vi "GetRotaryColorScaleReference.vi"(8 "error in":errorcluster, 11 "RotaryColorScale in":refnum<class "RotaryColorScale.lvclass">) -> (0 "error out":errorcluster, 1 "color scale reference":refnum<vi>, 3 "RotaryColorScale out":refnum<class "RotaryColorScale.lvclass">)   [LabVIEW 2014, in "Raspberry Pi Compatible Compiler for LabVIEW.lvlib" / "RotaryColorScale.lvclass"]
uses:
  RotaryColorScale.lvclass
  Generic/Generic.lvclass
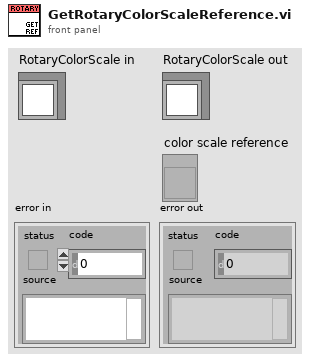
[diagram p1: front panel]
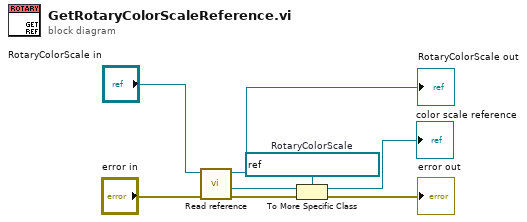
[diagram p0: block diagram]
diagram:
  w5 = refnum<vi> refnum  # RotaryColorScale
  n1 = call "Read reference.vi"("error in"="error in", "GObject in"="RotaryColorScale in") -> ("error out"=w6:errorcluster, "reference"=w7:refnum<vi>, "GObject out"=→"RotaryColorScale out":refnum<class "RotaryColorScale.lvclass">)  [unwired: 5 in]
  n2 = To More Specific Class(target class=w5, reference=w7, error in=w6) -> (specific class reference=→"color scale reference":refnum<vi>, error out=→"error out":errorcluster)
